vi "Read any file only.vi"(0 "Input file path":path, 1 "Trigger delay":i32, 2 "Data points":i32=-1, 5 "Data File Type":T1(ring)=enum."BinH File", 7 "number of header lines":i32, 9 "Ext Clock Freq":dbl format="%.2f", 11 "2D number of rows":i32, 12 "transpose (no:F)":bool=TRUE, 15 "2D number of columns/1D count (all as 1D: -1)":i32=1) -> (3 "Header":string, 4 "Actual input file path":path, 6 "all rows":sgl[][](array[numeric]) format="%.2e", 8 "Actual Delay":i32, 10 "Actual Rate":dbl format="%.2f", 13 "Delay, points":dbl format="%.2f", 14 "Time base":dbl format="%.2e")   [LabVIEW 2021]
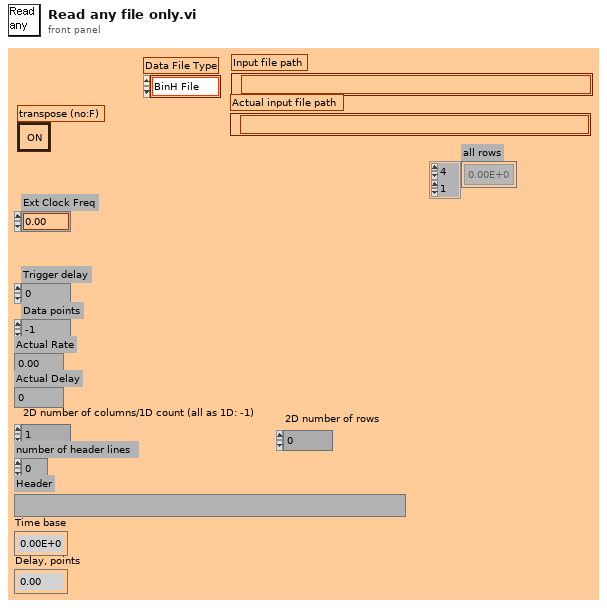
[diagram p1: front panel]
types:
  T1 = enum16{"ASCII File", "BinH File", "BinW File", "BINARY File"}
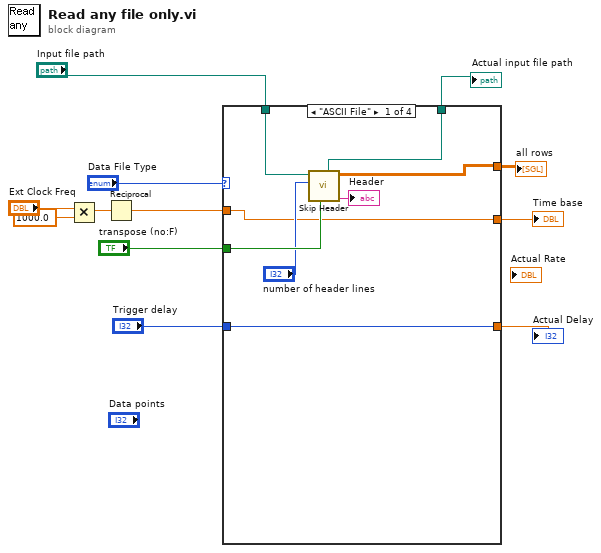
[diagram p0: block diagram]
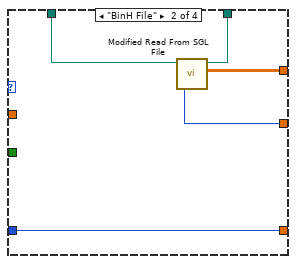
[diagram p2: hidden frame]
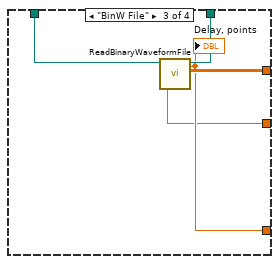
[diagram p3: hidden frame]
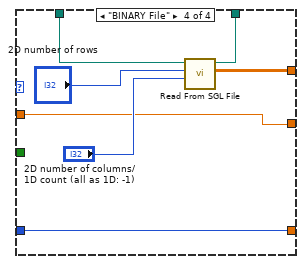
[diagram p4: hidden frame]
diagram:
  n1 = Multiply(x="Ext Clock Freq", y=1000.0) -> (x*y=w2:dbl)
  n2 = Reciprocal(x=w2) -> (1/x=w1:dbl)
  n3 = case shown="\"ASCII File\"" "Data File Type" {
    tunnel: "Input file path" -> [w20 w25 w30 w37]
    tunnel: [w19 w24 w29 w36] -> w10
    tunnel: [w18 w23 w28 w35] -> w8
    tunnel: "transpose (no:F)" -> [w17 _ _ _]
    tunnel: "Trigger delay" -> [w16 w22 _ w33]
    tunnel: [w16 w22 w27 w33] -> w6
    tunnel: [w13 w21 w26 w32] -> w5
    tunnel: w1 -> [w13 _ _ w32]
    frame "ASCII File" {
      n4 = call "Skip Header.vi"("transpose (yes:T)"=w17, "number of header lines"="number of header lines", "Input File Name"=w20) -> ("Header"=→"Header":string, "all rows"=w18:dbl[][], "new file path (Not A Path if cancelled)"=w19:path)  [unwired: 2 in, 4 out]
    }
    frame "BinH File" {
      n5 = call "Modified Read From SGL File.vi"("file path (dialog if empty)"=w25) -> ("2D array"=w23:sgl[][], "new file path (Not A Path if cancelled)"=w24:path, "mark after read (bytes)"=w21:i32)  [unwired: 2 in, 6 out]
    }
    frame "BinW File" {
      n6 = call "ReadBinaryWaveformFile.vi"("file path (dialog if empty)"=w30) -> ("2D array"=w28:sgl[][], "new file path (Not A Path if cancelled)"=w29:path, "Time base"=w26:dbl, "Delay, points"=w27:dbl)  [unwired: 2 in, 5 out]
      "Delay, points" <- w27
    }
    frame "BINARY File" {
      n7 = call <vilib>:"Read From SGL File.vi"("2D number of columns/1D count (all as 1D: -1)"="2D number of columns/1D count (all as 1D: -1)", "2D number of rows"="2D number of rows", "file path (dialog if empty)"=w37) -> ("2D array"=w35:sgl[][], "new file path (Not A Path if cancelled)"=w36:path)  [unwired: 7 out]
    }
  }
  "Actual input file path" <- w10
  "all rows" <- w8
  "Actual Delay" <- w6
  "Time base" <- w5
